vi "checkFirstTimestamp.vi"(8 "error in (no error)":errorcluster, 11 "GuassianNoiseWave in":refnum<class "GuassianNoiseWave.lvclass">) -> (0 "error out":errorcluster, 2 "IsFirst":bool, 3 "GuassianNoiseWave out":refnum<class "GuassianNoiseWave.lvclass">)   [LabVIEW 2015, in "GuassianNoiseWave.lvclass"]
uses:
  GuassianNoiseWave.lvclass
  GuassianNoiseWave.lvclass/GuassianNoiseWave.ctl
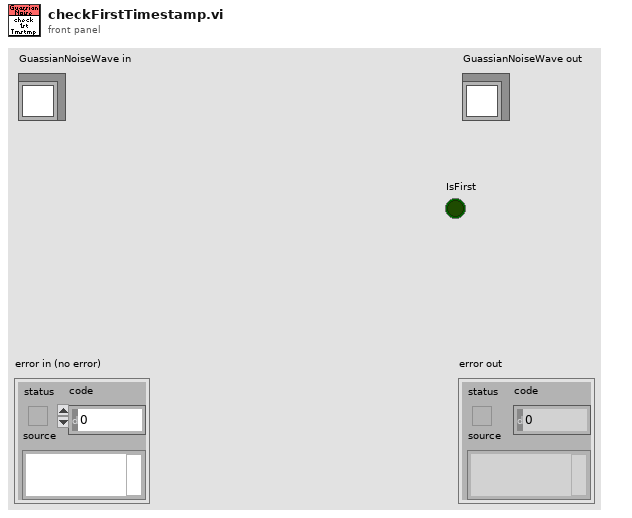
[diagram p1: front panel]
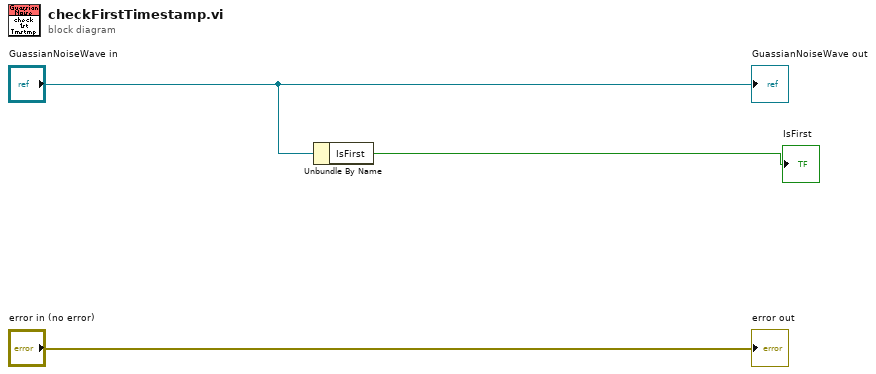
[diagram p0: block diagram]
diagram:
  n1 = Unbundle By Name("GuassianNoiseWave in") -> ("IsFirst"=→"IsFirst":bool)
  "error out" <- "error in (no error)"
  "GuassianNoiseWave out" <- "GuassianNoiseWave in"
